vi "ROI_Image_Draw Feret Line.vi"(6 "Pixel Measurements":T4[](array[typedef]) items=["Center of Mass X", "Center of Mass Y", "First Pixel X", "First Pixel Y", "Bounding Rect Left", "Bounding Rect Top", "Bounding Rect Right", "Bounding Rect Bottom", "Max Feret Diameter Start X", "Max Feret Diameter Start Y", "Max Feret Diameter End X", "Max Feret Diameter End Y", "Max Horiz. Segment Length Left", "Max Horiz. Segment Length Right", "Max Horiz. Segment Length Row", "-", "Bounding Rect Width", "Bounding Rect Height", "Bounding Rect Diagonal", "Perimeter", "Convex Hull Perimeter", "Holes' Perimeter", "Max Feret Diameter", "Equivalent Ellipse Major Axis", "Equivalent Ellipse Minor Axis", "Equivalent Ellipse Minor Axis (Feret)", "Equivalent Rect Long Side", "Equivalent Rect Short Side", "Equivalent Rect Diagonal", "Equivalent Rect Short Side (Feret)", "Average Horiz. Segment Length", "Average Vert. Segment Length", "Hydraulic Radius", "Waddel Disk Diameter", "-", "Area", "Holes' Area", "Particle & Holes' Area", "Convex Hull Area", "Image Area", "-", "Number of Holes", "Number of Horiz. Segments", "Number of Vert. Segments", "-", "Orientation", "Max Feret Diameter Orientation", "-", "% Area/Image Area", "% Area/(Particle & Holes' Area)", "Ratio of Equivalent Ellipse Axes", "Ratio of Equivalent Rect Sides", "-", "Elongation Factor", "Compactness Factor", "Heywood Circularity Factor", "Type Factor", "-", "Sum X", "Sum Y", "Sum XX", "Sum XY", "Sum YY", "Sum XXX", "Sum XXY", "Sum XYY", "Sum YYY", "-", "Moment of Inertia XX", "Moment of Inertia XY", "Moment of Inertia YY", "Moment of Inertia XXX", "Moment of Inertia XXY", "Moment of Inertia XYY", "Moment of Inertia YYY", "Norm. Moment of Inertia XX", "Norm. Moment of Inertia XY", "Norm. Moment of Inertia YY", "Norm. Moment of Inertia XXX", "Norm. Moment of Inertia XXY", "Norm. Moment of Inertia XYY", "Norm. Moment of Inertia YYY", "Hu Moment 1", "Hu Moment 2", "Hu Moment 3", "Hu Moment 4", "Hu Moment 5", "Hu Moment 6", "Hu Moment 7"], 8 "error in (no error)":errorcluster, 9 "Particle Measurements (Pixels)":dbl[][](array[numeric]), 10 "Circles Data":T3(array[cluster]), 11 "Image in":T1) -> (0 "error out":errorcluster, 2 "ROI":T2 {"Contours"."Type" items=["No Selection", "Point", "Line", "Rectangle", "Oval", "Polygon", "Freehand Region", "Annulus", "Unused2", "Unused3", "Broken Line", "Freehand Line", "Rotated Rectangle"]}, 3 "Image out":T1)   [LabVIEW 2012]
uses:
  <vilib>/vision/Image Controls.llb/IMAQ Image.ctl
  <vilib>/vision/NI_Vision_Development_Module.lvlib
panel:
  out "Image for display":T1(plugin-control)
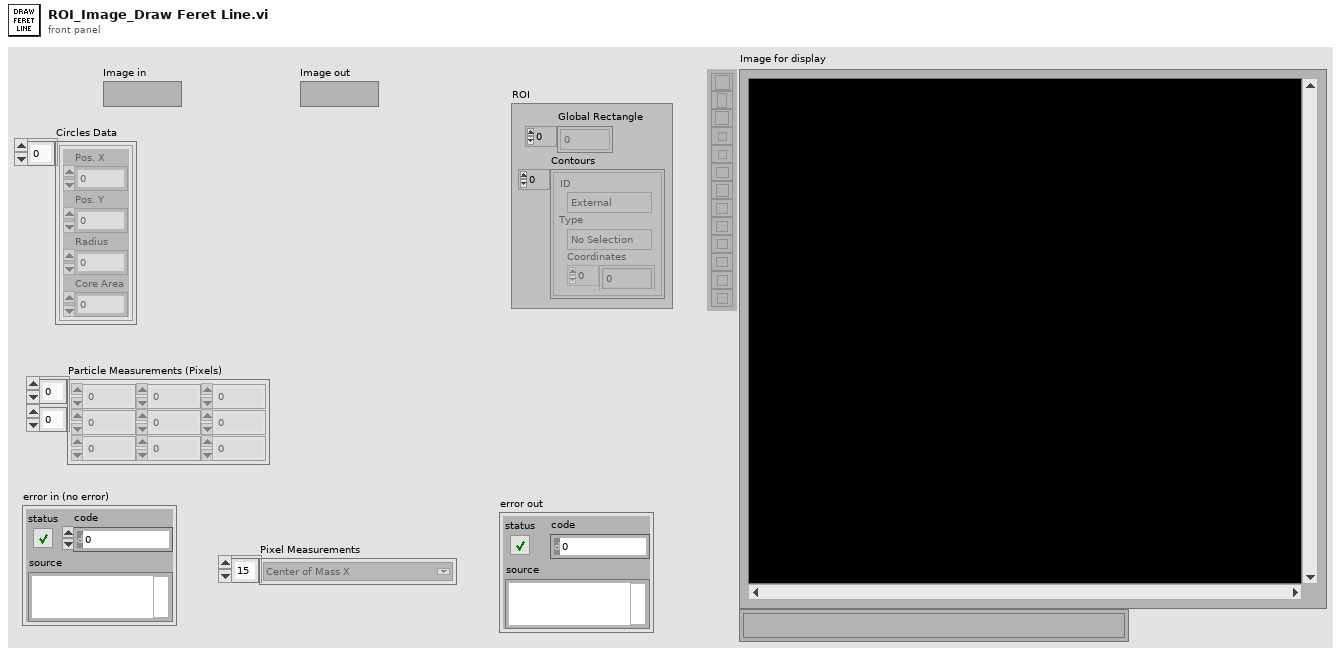
[diagram p1: front panel]
types:
  T1 = typedef "IMAQ Image.ctl" = refnum<image>
  T2 = typedef "ROI Descriptor" = cluster{"Global Rectangle":i32[], "Contours":cluster{"ID":enum32{"External", "Internal"}, "Type":u32, "Coordinates":i32[]}[]}
  T3 = cluster{"Pos. X":i32, "Pos. Y":i32, "Radius":i32, "Core Area":i32}[]
  T4 = typedef "Particle Parameters" = i32
  T5 = cluster{"Left":i32, "Top":i32, "Right":i32, "Bottom":i32}
  T6 = cluster{"Pos. X":i32, "Pos. Y":i32, "Radius":i32, "Core Area":i32}
  T7 = typedef "enum - StartPt Relative to Circle Center.ctl" = enum16{"X to the Right; Y Below", "X to the Right; Y Above", "X to the Left; Y Below", "X to the Left: Y Above"}
  T8 = cluster{"Point 1":cluster{"X":sgl, "Y":sgl}, "Point 2":cluster{"X":sgl, "Y":sgl}}
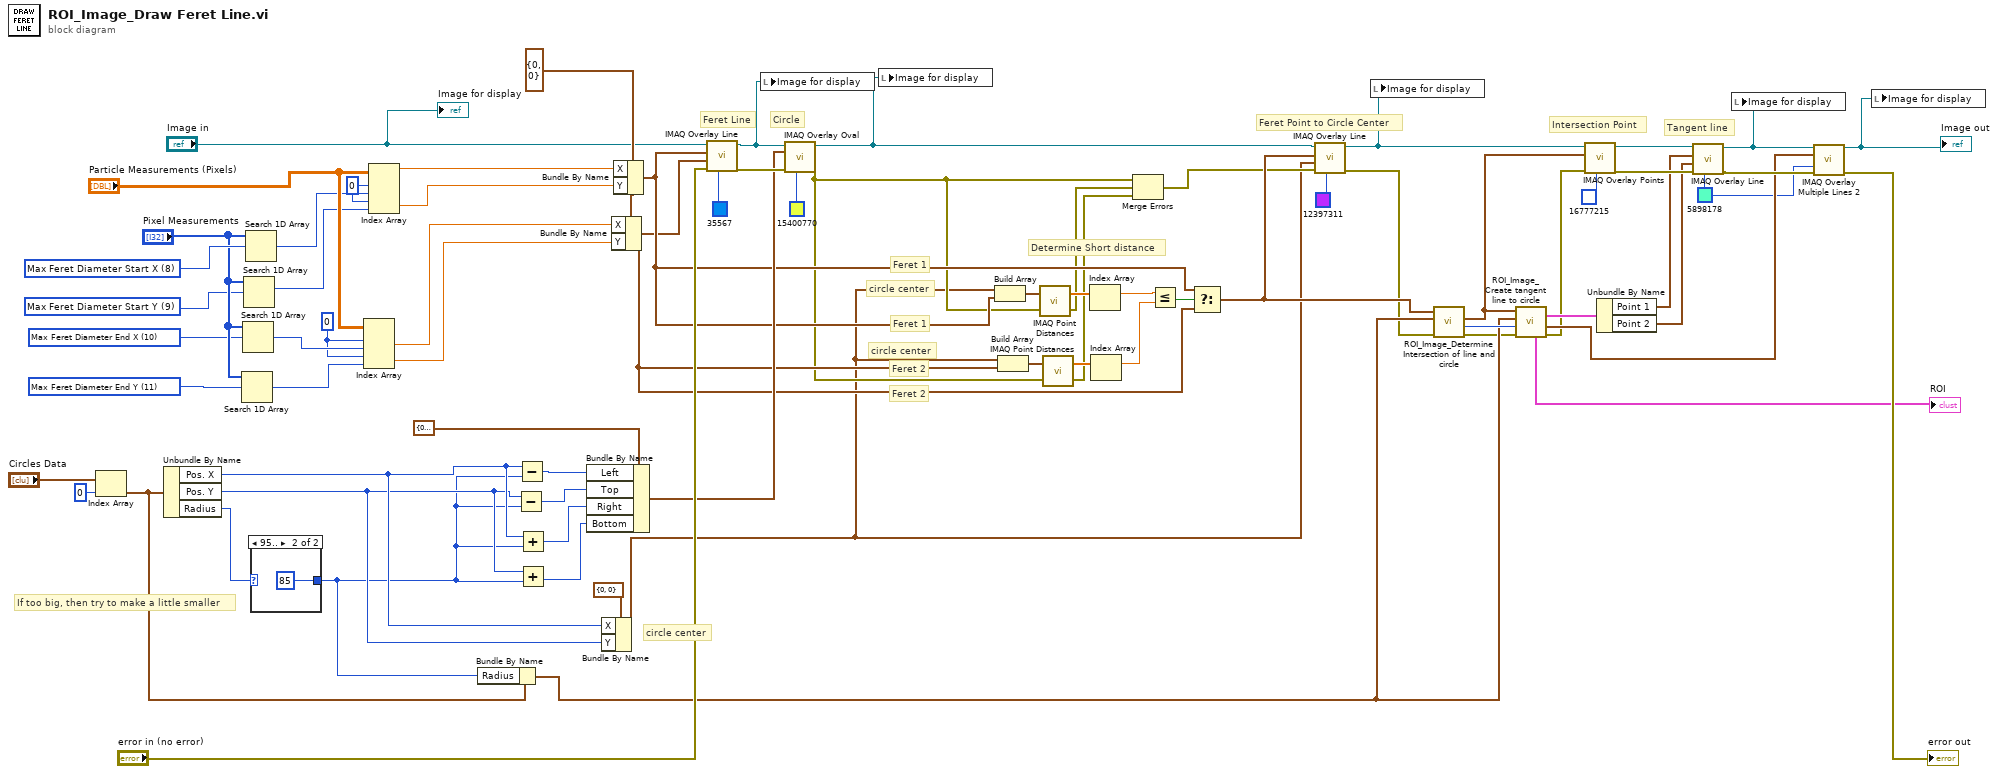
[diagram p0: block diagram]
diagram:
  w23 = u32 5898178 ("Color")
  w57 = 0 ("disabled index (col)")
  w61 = 0 ("disabled index (col)")
  w74 = cluster{"X":i32, "Y":i32} {"X"=0, "Y"=0} ("Start Point")
  w69 = T4 11 items=["Center of Mass X", "Center of Mass Y", "First Pixel X", "First Pixel Y", "Bounding Rect Left", "Bounding Rect Top", "Bounding Rect Right", "Bounding Rect Bottom", "Max Feret Diameter Start X", "Max Feret Diameter Start Y", "Max Feret Diameter End X", "Max Feret Diameter End Y", "Max Horiz. Segment Length Left", "Max Horiz. Segment Length Right", "Max Horiz. Segment Length Row", "-", "Bounding Rect Width", "Bounding Rect Height", "Bounding Rect Diagonal", "Perimeter", "Convex Hull Perimeter", "Holes' Perimeter", "Max Feret Diameter", "Equivalent Ellipse Major Axis", "Equivalent Ellipse Minor Axis", "Equivalent Ellipse Minor Axis (Feret)", "Equivalent Rect Long Side", "Equivalent Rect Short Side", "Equivalent Rect Diagonal", "Equivalent Rect Short Side (Feret)", "Average Horiz. Segment Length", "Average Vert. Segment Length", "Hydraulic Radius", "Waddel Disk Diameter", "-", "Area", "Holes' Area", "Particle & Holes' Area", "Convex Hull Area", "Image Area", "-", "Number of Holes", "Number of Horiz. Segments", "Number of Vert. Segments", "-", "Orientation", "Max Feret Diameter Orientation", "-", "% Area/Image Area", "% Area/(Particle & Holes' Area)", "Ratio of Equivalent Ellipse Axes", "Ratio of Equivalent Rect Sides", "-", "Elongation Factor", "Compactness Factor", "Heywood Circularity Factor", "Type Factor", "-", "Sum X", "Sum Y", "Sum XX", "Sum XY", "Sum YY", "Sum XXX", "Sum XXY", "Sum XYY", "Sum YYY", "-", "Moment of Inertia XX", "Moment of Inertia XY", "Moment of Inertia YY", "Moment of Inertia XXX", "Moment of Inertia XXY", "Moment of Inertia XYY", "Moment of Inertia YYY", "Norm. Moment of Inertia XX", "Norm. Moment of Inertia XY", "Norm. Moment of Inertia YY", "Norm. Moment of Inertia XXX", "Norm. Moment of Inertia XXY", "Norm. Moment of Inertia XYY", "Norm. Moment of Inertia YYY", "Hu Moment 1", "Hu Moment 2", "Hu Moment 3", "Hu Moment 4", "Hu Moment 5", "Hu Moment 6", "Hu Moment 7"] ("Measurement Parameter")
  w70 = T4 10 items=["Center of Mass X", "Center of Mass Y", "First Pixel X", "First Pixel Y", "Bounding Rect Left", "Bounding Rect Top", "Bounding Rect Right", "Bounding Rect Bottom", "Max Feret Diameter Start X", "Max Feret Diameter Start Y", "Max Feret Diameter End X", "Max Feret Diameter End Y", "Max Horiz. Segment Length Left", "Max Horiz. Segment Length Right", "Max Horiz. Segment Length Row", "-", "Bounding Rect Width", "Bounding Rect Height", "Bounding Rect Diagonal", "Perimeter", "Convex Hull Perimeter", "Holes' Perimeter", "Max Feret Diameter", "Equivalent Ellipse Major Axis", "Equivalent Ellipse Minor Axis", "Equivalent Ellipse Minor Axis (Feret)", "Equivalent Rect Long Side", "Equivalent Rect Short Side", "Equivalent Rect Diagonal", "Equivalent Rect Short Side (Feret)", "Average Horiz. Segment Length", "Average Vert. Segment Length", "Hydraulic Radius", "Waddel Disk Diameter", "-", "Area", "Holes' Area", "Particle & Holes' Area", "Convex Hull Area", "Image Area", "-", "Number of Holes", "Number of Horiz. Segments", "Number of Vert. Segments", "-", "Orientation", "Max Feret Diameter Orientation", "-", "% Area/Image Area", "% Area/(Particle & Holes' Area)", "Ratio of Equivalent Ellipse Axes", "Ratio of Equivalent Rect Sides", "-", "Elongation Factor", "Compactness Factor", "Heywood Circularity Factor", "Type Factor", "-", "Sum X", "Sum Y", "Sum XX", "Sum XY", "Sum YY", "Sum XXX", "Sum XXY", "Sum XYY", "Sum YYY", "-", "Moment of Inertia XX", "Moment of Inertia XY", "Moment of Inertia YY", "Moment of Inertia XXX", "Moment of Inertia XXY", "Moment of Inertia XYY", "Moment of Inertia YYY", "Norm. Moment of Inertia XX", "Norm. Moment of Inertia XY", "Norm. Moment of Inertia YY", "Norm. Moment of Inertia XXX", "Norm. Moment of Inertia XXY", "Norm. Moment of Inertia XYY", "Norm. Moment of Inertia YYY", "Hu Moment 1", "Hu Moment 2", "Hu Moment 3", "Hu Moment 4", "Hu Moment 5", "Hu Moment 6", "Hu Moment 7"] ("Measurement Parameter")
  w71 = T4 9 items=["Center of Mass X", "Center of Mass Y", "First Pixel X", "First Pixel Y", "Bounding Rect Left", "Bounding Rect Top", "Bounding Rect Right", "Bounding Rect Bottom", "Max Feret Diameter Start X", "Max Feret Diameter Start Y", "Max Feret Diameter End X", "Max Feret Diameter End Y", "Max Horiz. Segment Length Left", "Max Horiz. Segment Length Right", "Max Horiz. Segment Length Row", "-", "Bounding Rect Width", "Bounding Rect Height", "Bounding Rect Diagonal", "Perimeter", "Convex Hull Perimeter", "Holes' Perimeter", "Max Feret Diameter", "Equivalent Ellipse Major Axis", "Equivalent Ellipse Minor Axis", "Equivalent Ellipse Minor Axis (Feret)", "Equivalent Rect Long Side", "Equivalent Rect Short Side", "Equivalent Rect Diagonal", "Equivalent Rect Short Side (Feret)", "Average Horiz. Segment Length", "Average Vert. Segment Length", "Hydraulic Radius", "Waddel Disk Diameter", "-", "Area", "Holes' Area", "Particle & Holes' Area", "Convex Hull Area", "Image Area", "-", "Number of Holes", "Number of Horiz. Segments", "Number of Vert. Segments", "-", "Orientation", "Max Feret Diameter Orientation", "-", "% Area/Image Area", "% Area/(Particle & Holes' Area)", "Ratio of Equivalent Ellipse Axes", "Ratio of Equivalent Rect Sides", "-", "Elongation Factor", "Compactness Factor", "Heywood Circularity Factor", "Type Factor", "-", "Sum X", "Sum Y", "Sum XX", "Sum XY", "Sum YY", "Sum XXX", "Sum XXY", "Sum XYY", "Sum YYY", "-", "Moment of Inertia XX", "Moment of Inertia XY", "Moment of Inertia YY", "Moment of Inertia XXX", "Moment of Inertia XXY", "Moment of Inertia XYY", "Moment of Inertia YYY", "Norm. Moment of Inertia XX", "Norm. Moment of Inertia XY", "Norm. Moment of Inertia YY", "Norm. Moment of Inertia XXX", "Norm. Moment of Inertia XXY", "Norm. Moment of Inertia XYY", "Norm. Moment of Inertia YYY", "Hu Moment 1", "Hu Moment 2", "Hu Moment 3", "Hu Moment 4", "Hu Moment 5", "Hu Moment 6", "Hu Moment 7"] ("Measurement Parameter")
  w73 = T4 8 items=["Center of Mass X", "Center of Mass Y", "First Pixel X", "First Pixel Y", "Bounding Rect Left", "Bounding Rect Top", "Bounding Rect Right", "Bounding Rect Bottom", "Max Feret Diameter Start X", "Max Feret Diameter Start Y", "Max Feret Diameter End X", "Max Feret Diameter End Y", "Max Horiz. Segment Length Left", "Max Horiz. Segment Length Right", "Max Horiz. Segment Length Row", "-", "Bounding Rect Width", "Bounding Rect Height", "Bounding Rect Diagonal", "Perimeter", "Convex Hull Perimeter", "Holes' Perimeter", "Max Feret Diameter", "Equivalent Ellipse Major Axis", "Equivalent Ellipse Minor Axis", "Equivalent Ellipse Minor Axis (Feret)", "Equivalent Rect Long Side", "Equivalent Rect Short Side", "Equivalent Rect Diagonal", "Equivalent Rect Short Side (Feret)", "Average Horiz. Segment Length", "Average Vert. Segment Length", "Hydraulic Radius", "Waddel Disk Diameter", "-", "Area", "Holes' Area", "Particle & Holes' Area", "Convex Hull Area", "Image Area", "-", "Number of Holes", "Number of Horiz. Segments", "Number of Vert. Segments", "-", "Orientation", "Max Feret Diameter Orientation", "-", "% Area/Image Area", "% Area/(Particle & Holes' Area)", "Ratio of Equivalent Ellipse Axes", "Ratio of Equivalent Rect Sides", "-", "Elongation Factor", "Compactness Factor", "Heywood Circularity Factor", "Type Factor", "-", "Sum X", "Sum Y", "Sum XX", "Sum XY", "Sum YY", "Sum XXX", "Sum XXY", "Sum XYY", "Sum YYY", "-", "Moment of Inertia XX", "Moment of Inertia XY", "Moment of Inertia YY", "Moment of Inertia XXX", "Moment of Inertia XXY", "Moment of Inertia XYY", "Moment of Inertia YYY", "Norm. Moment of Inertia XX", "Norm. Moment of Inertia XY", "Norm. Moment of Inertia YY", "Norm. Moment of Inertia XXX", "Norm. Moment of Inertia XXY", "Norm. Moment of Inertia XYY", "Norm. Moment of Inertia YYY", "Hu Moment 1", "Hu Moment 2", "Hu Moment 3", "Hu Moment 4", "Hu Moment 5", "Hu Moment 6", "Hu Moment 7"] ("Measurement Parameter")
  # "Feret 1"
  # "Feret 2"
  # "circle center"
  # "Feret 2"
  # "Feret 1"
  # "circle center"
  # "circle center"
  # "If too big, then try to make a little smaller"
  # "Tangent line"
  # "Feret Point to Circle Center"
  # "Determine Short distance"
  # "Intersection Point"
  # "Circle"
  # "Feret Line"
  n1 = Index Array(array="Circles Data", index=0) -> (element=w20:T6)
  n2 = Unbundle By Name(w20) -> ("Pos. X"=w45:i32, "Pos. Y"=w44:i32, "Radius"=w18:i32)
  n3 = Search 1D Array(1D array="Pixel Measurements", element=w69) -> (index of element=w56:i32)  [unwired: 1 in]
  n4 = Search 1D Array(1D array="Pixel Measurements", element=w70) -> (index of element=w58:i32)  [unwired: 1 in]
  n5 = Search 1D Array(1D array="Pixel Measurements", element=w71) -> (index of element=w59:i32)  [unwired: 1 in]
  n6 = Search 1D Array(1D array="Pixel Measurements", element=w73) -> (index of element=w60:i32)  [unwired: 1 in]
  n7 = case shown="95.." w18 {
    selector: w18 -> [w75 _]
    tunnel: [w75 85 ("y")] -> w17
    frame 0, Default {
    }
    frame 95.. {
    }
  }
  n8 = Index Array(array="Particle Measurements (Pixels)", index (row) #1=w57, index (col) #1=w58, index (row) #2=w57, index (col) #2=w56) -> (element #1=w65:dbl, element #2=w64:dbl)
  n9 = Index Array(array="Particle Measurements (Pixels)", index (row) #1=w61, index (col) #1=w60, index (row) #2=w61, index (col) #2=w59) -> (element #1=w68:dbl, element #2=w67:dbl)
  n10 = Bundle By Name(cluster=w20, "Radius"=w17) -> (w19:T6)
  n11 = Subtract(x=w44, y=w17) -> (x-y=w51:i32)
  n12 = Subtract(x=w45, y=w17) -> (x-y=w52:i32)
  n13 = Add(x=w45, y=w17) -> (x+y=w50:i32)
  n14 = Add(x=w44, y=w17) -> (x+y=w49:i32)
  n15 = Bundle By Name(cluster=T5 {"Left"=0, "Top"=0, "Right"=0, "Bottom"=0} ("Bounding Rectangle"), "Left"=w52, "Top"=w51, "Right"=w50, "Bottom"=w49) -> (w48:T5)
  n16 = Bundle By Name(cluster=cluster{"X":i32, "Y":i32} {"X"=0, "Y"=0} ("Point"), "X"=w45, "Y"=w44) -> (w1:cluster{"X":i32, "Y":i32})
  n17 = Bundle By Name(cluster=w74, "X"=w65, "Y"=w64) -> (w35:cluster{"X":i32, "Y":i32})
  n18 = Bundle By Name(cluster=w74, "X"=w68, "Y"=w67) -> (w36:cluster{"X":i32, "Y":i32})
  n19 = call "IMAQ Overlay Line"("Color"=u32 35567, "error in (no error)"="error in (no error)", "End Point"=w35, "Start Point"=w36, "Image"="Image in") -> ("error out"=w55:errorcluster, "Image Out"=w8:T1)  [unwired: 5 in]
  n20 = local write "Image for display"(w8) -> ()
  n21 = call "IMAQ Overlay Oval"("Color"=u32 15400770, "error in (no error)"=w55, "Bounding Rectangle"=w48, "Image"=w8) -> ("error out"=w16:errorcluster, "Image Out"=w7:T1)  [unwired: 6 in]
  n22 = local write "Image for display"(w7) -> ()
  n23 = Build Array(w1, w36) -> (w43:cluster{"X":i32, "Y":i32}[])
  n24 = Build Array(w1, w35) -> (w42:cluster{"X":i32, "Y":i32}[])
  n25 = call "IMAQ Point Distances"("Points"=w43, "error in (no error)"=w16) -> ("Distances"=w41:sgl[], "error out"=w12:errorcluster)  [unwired: 3 in]
  n26 = call "IMAQ Point Distances"("Points"=w42, "error in (no error)"=w16) -> ("Distances"=w40:sgl[], "error out"=w11:errorcluster)  [unwired: 3 in]
  n27 = Index Array(array=w41) -> (element=w39:sgl)  [unwired: 1 in]
  n28 = Index Array(array=w40) -> (element=w38:sgl)  [unwired: 1 in]
  n29 = Merge Errors(w16, w12, w11) -> (w13:errorcluster)
  n30 = Less Or Equal?(x=w39, y=w38) -> (x <= y?=w37:bool)
  n31 = Select(t=w36, s=w37, f=w35) -> (s? t:f=w33:cluster{"X":i32, "Y":i32})
  n32 = call "IMAQ Overlay Line"("Color"=u32 12397311, "error in (no error)"=w13, "End Point"=w1, "Start Point"=w33, "Image"=w7) -> ("error out"=w3:errorcluster, "Image Out"=w6:T1)  [unwired: 5 in]
  n33 = local write "Image for display"(w6) -> ()
  n34 = call "ROI_Image_Determine Intersection of line and circle.vi"("error in (no error)"=w3, "Circles Data"=w19, "Start Point"=w33) -> ("error out"=w15:errorcluster, "Orient rel to center"=w22:T7, "Intersection point"=w10:cluster{"X":i32, "Y":i32})  [unwired: 6 in]
  n35 = call "ROI_Image_Create tangent line to circle.vi"("error in (no error)"=w15, "Orient rel to center"=w22, "Circles Data"=w19, "Intersection Point"=w10) -> ("error out"=w14:errorcluster, "Line End Points"=w24:cluster{"X":dbl, "Y":dbl}[], "Tangent Line"=w29:T8, "ROI"=→"ROI":T2)  [unwired: 4 in]
  n36 = call "IMAQ Overlay Points"("Color"=u32 16777215, "error in (no error)"=w14, "Point"=w10, "Image"=w6) -> ("error out"=w31:errorcluster, "Image Out"=w30:T1)  [unwired: 6 in]
  n37 = Unbundle By Name(w29) -> ("Point 1"=w28:cluster{"X":sgl, "Y":sgl}, "Point 2"=w27:cluster{"X":sgl, "Y":sgl})
  n38 = call "IMAQ Overlay Line"("Color"=w23, "error in (no error)"=w31, "End Point"=w27, "Start Point"=w28, "Image"=w30) -> ("error out"=w26:errorcluster, "Image Out"=w5:T1)  [unwired: 5 in]
  n39 = local write "Image for display"(w5) -> ()
  n40 = call "IMAQ Overlay Multiple Lines 2"("Image"=w5, "Line End Points"=w24, "Color"=w23, "error in (no error)"=w26) -> ("Image Out"=w4:T1, "error out"=→"error out":errorcluster)  [unwired: 10 in]
  "Image out" <- w4
  n41 = local write "Image for display"(w4) -> ()
  "Image for display" <- "Image in"
